vi "SupportedFunctions.vi"(11 "Functions":T1=[{"module"="pyVI.FP.lvFrontPanel", "short name"="", "docstrings"={"type"="def", "name"="_async_raise", "docstring"="raises the exception, performs cleanup if needed"}}, {"module"="pyVI.FP.lvFrontPanel", "short name"="", "docstrings"={"type"="def", "name"="_get_my_tid", "docstring"="determines this (self's) thread id"}}, {"module"="pyVI.FP.lvFrontPanel", "short name"="", "docstrings"={"type"="def", "name"="raise_exc", "docstring"="raises the given exception type in the context of this thread"}}, {"module"="pyVI.FP.lvFrontPanel", "short name"="", "docstrings"={"type"="def", "name"="terminate", "docstring"="raises SystemExit in the context of the given thread, which should \r\n        cause the thread to exit silently (unless caught)"}}, {"module"="pyVI.functions.lvAdvancedFileFunctions", "short name"="lvAdvFile", "docstrings"={"type"="class", "name"="GetFilePosition", "docstring"="_LV_(Get File Position,[1,0],[2,1,0])"}}, {"module"="pyVI.functions.lvAdvancedFileFunctions", "short name"="lvAdvFile", "docstrings"={"type"="class", "name"="GetFileSize", "docstring"="_LV_(Get File Size,[1,0],[2,1,0])"}}, {"module"="pyVI.functions.lvAdvancedFileFunctions", "short name"="lvAdvFile", "docstrings"={"type"="class", "name"="SetFileSize", "docstring"="_LV_(Set File Size,[2,1,0],[1,0])"}}, {"module"="pyVI.functions.lvAdvancedFileFunctions", "short name"="lvAdvFile", "docstrings"={"type"="class", "name"="SetFilePosition", "docstring"="_LV_(Set File Position,[3,2,1,0],[1,0])"}}, {"module"="pyVI.functions.lvAdvancedFileFunctions", "short name"="lvAdvFile", "docstrings"={"type"="class", "name"="MoveFile", "docstring"="_LV_(Move,[4,3,2,0,1],[2,1,0])"}}, {"module"="pyVI.functions.lvAdvancedFileFunctions", "short name"="lvAdvFile", "docstrings"={"type"="class", "name"="CopyFile", "docstring"="_LV_(Copy,[4,3,2,0,1],[2,1,0])"}}, {"module"="pyVI.functions.lvAdvancedFileFunctions", "short name"="lvAdvFile", "docstrings"={"type"="class", "name"="DeleteFile", "docstring"="_LV_(Delete,[4,3,2,0,1],[2,1,0])"}}, {"module"="pyVI.functions.lvAdvancedFileFunctions", "short name"="lvAdvFile", "docstrings"={"type"="class", "name"="CreateFolder", "docstring"="_LV_(Create Folder,[2,0,1],[2,1,0])"}}, {"module"="pyVI.functions.lvAdvancedFileFunctions", "short name"="lvAdvFile", "docstrings"={"type"="class", "name"="ListFolder", "docstring"="_LV_(List Folder,[3,1,0,2],[3,2,1,0])"}}, {"module"="pyVI.functions.lvAdvancedFileFunctions", "short name"="lvAdvFile", "docstrings"={"type"="class", "name"="RefnumToPath", "docstring"="_LV_(Refnum to Path,[0],[0])"}}, {"module"="pyVI.functions.lvAdvancedFileFunctions", "short name"="lvAdvFile", "docstrings"={"type"="class", "name"="PathType", "docstring"="_LV_(Path Type,[0],[0])"}}, {"module"="pyVI.functions.lvArrayFunctions", "short name"="lvArray", "docstrings"={"type"="class", "name"="BuildArray", "docstring"="_LV_(Build Array,[0..],[0])"}}, {"module"="pyVI.functions.lvArrayFunctions", "short name"="lvArray", "docstrings"={"type"="class", "name"="IndexArray", "docstring"="_LV_(Index Array,[0,1..],[0..])"}}, {"module"="pyVI.functions.lvArrayFunctions", "short name"="lvArray", "docstrings"={"type"="class", "name"="ArraySize", "docstring"="_LV_(Array Size,[0],[0])"}}, {"module"="pyVI.functions.lvArrayFunctions", "short name"="lvArray", "docstrings"={"type"="class", "name"="InitializeArray", "docstring"="_LV_(Initialize Array,[0,1..],[0])"}}, {"module"="pyVI.functions.lvArrayFunctions", "short name"="lvArray", "docstrings"={"type"="class", "name"="ArraySubset", "docstring"="_LV_(Array Subset,[0,1,2..],[0])"}}, {"module"="pyVI.functions.lvArrayFunctions", "short name"="lvArray", "docstrings"={"type"="class", "name"="ArrayMaxMin", "docstring"="_LV_(Array Max & Min,[0],[0,1,2,3])"}}, {"module"="pyVI.functions.lvArrayFunctions", "short name"="lvArray", "docstrings"={"type"="class", "name"="ReshapeArray", "docstring"="_LV_(Reshape Array,[0,1..],[0])"}}, {"module"="pyVI.functions.lvArrayFunctions", "short name"="lvArray", "docstrings"={"type"="class", "name"="SortArray", "docstring"="_LV_(Sort 1D Array,[0],[0])"}}, {"module"="pyVI.functions.lvArrayFunctions", "short name"="lvArray", "docstrings"={"type"="class", "name"="SearchArray", "docstring"="_LV_(Search 1D Array,[2,1,0],[0])"}}, {"module"="pyVI.functions.lvArrayFunctions", "short name"="lvArray", "docstrings"={"type"="class", "name"="SplitArray", "docstring"="_LV_(Split 1D Array,[1,0],[1,0])"}}, {"module"="pyVI.functions.lvArrayFunctions", "short name"="lvArray", "docstrings"={"type"="class", "name"="ReverseArray", "docstring"="_LV_(Reverse 1D Array,[0],[0])"}}, {"module"="pyVI.functions.lvArrayFunctions", "short name"="lvArray", "docstrings"={"type"="class", "name"="RotateArray", "docstring"="_LV_(Rotate 1D Array,[0,1],[0])"}}, {"module"="pyVI.functions.lvArrayFunctions", "short name"="lvArray", "docstrings"={"type"="class", "name"="InterleaveArrays", "docstring"="_LV_(Interleave 1D Arrays,[0..],[0])"}}, {"module"="pyVI.functions.lvArrayFunctions", "short name"="lvArray", "docstrings"={"type"="class", "name"="DecimateArray", "docstring"="_LV_(Decimate 1D Array,[0],[0..])"}}, {"module"="pyVI.functions.lvArrayFunctions", "short name"="lvArray", "docstrings"={"type"="class", "name"="TransposeArray", "docstring"="_LV_(Transpose 2D Array,[0],[0])"}}, {"module"="pyVI.functions.lvArrayFunctions", "short name"="lvArray", "docstrings"={"type"="class", "name"="DeleteFromArray", "docstring"="_LV_(Delete From Array,[0,1,2..],[1,0])"}}, {"module"="pyVI.functions.lvArrayFunctions", "short name"="lvArray", "docstrings"={"type"="class", "name"="ReplaceArraySubset", "docstring"="_LV_(Replace Array Subset,[0,1,2..],[0])"}}, {"module"="pyVI.functions.lvArrayFunctions", "short name"="lvArray", "docstrings"={"type"="class", "name"="AddArrayElements", "docstring"="_LV_(Add Array Elements,[0],[0])"}}, {"module"="pyVI.functions.lvArrayFunctions", "short name"="lvArray", "docstrings"={"type"="class", "name"="MultiplyArrayElements", "docstring"="_LV_(Multiply Array Elements,[0],[0])"}}, {"module"="pyVI.functions.lvArrayFunctions", "short name"="lvArray", "docstrings"={"type"="class", "name"="Threshold1DArray", "docstring"="_LV_(Threshold 1D Array,[2,1,0],[0])"}}, {"module"="pyVI.functions.lvArrayFunctions", "short name"="lvArray", "docstrings"={"type"="class", "name"="Interpolate1DArray", "docstring"="_LV_(Interpolate 1D Array,[1,0],[0])"}}, {"module"="pyVI.functions.lvBooleanFunctions", "short name"="lvBool", "docstrings"={"type"="class", "name"="And", "docstring"="_LV_(And,[1,0],[0])"}}, {"module"="pyVI.functions.lvBooleanFunctions", "short name"="lvBool", "docstrings"={"type"="class", "name"="Or", "docstring"="_LV_(Or,[1,0],[0])"}}, {"module"="pyVI.functions.lvBooleanFunctions", "short name"="lvBool", "docstrings"={"type"="class", "name"="Xor", "docstring"="_LV_(Exclusive Or,[1,0],[0])"}}, {"module"="pyVI.functions.lvBooleanFunctions", "short name"="lvBool", "docstrings"={"type"="class", "name"="Not", "docstring"="_LV_(Not,[0],[0])"}}, {"module"="pyVI.functions.lvBooleanFunctions", "short name"="lvBool", "docstrings"={"type"="class", "name"="Nand", "docstring"="_LV_(Not And,[1,0],[0])"}}, {"module"="pyVI.functions.lvBooleanFunctions", "short name"="lvBool", "docstrings"={"type"="class", "name"="Nor", "docstring"="_LV_(Not Or,[1,0],[0])"}}, {"module"="pyVI.functions.lvBooleanFunctions", "short name"="lvBool", "docstrings"={"type"="class", "name"="Nxor", "docstring"="_LV_(Not Exclusive Or,[1,0],[0])"}}, {"module"="pyVI.functions.lvBooleanFunctions", "short name"="lvBool", "docstrings"={"type"="class", "name"="Implies", "docstring"="_LV_(Implies,[1,0],[0])"}}, {"module"="pyVI.functions.lvBooleanFunctions", "short name"="lvBool", "docstrings"={"type"="class", "name"="And_array_elements", "docstring"="_LV_(And Array Elements,[0],[0])"}}, {"module"="pyVI.functions.lvBooleanFunctions", "short name"="lvBool", "docstrings"={"type"="class", "name"="Or_array_elements", "docstring"="_LV_(Or Array Elements,[0],[0])"}}, {"module"="pyVI.functions.lvBooleanFunctions", "short name"="lvBool", "docstrings"={"type"="class", "name"="Number_to_boolean_array", "docstring"="_LV_(Number To Boolean Array,[0],[0])"}}, {"module"="pyVI.functions.lvBooleanFunctions", "short name"="lvBool", "docstrings"={"type"="class", "name"="Boolean_to_0_1", "docstring"="_LV_(Boolean To (0,1),[0],[0])"}}, {"module"="pyVI.functions.lvClusterFunctions", "short name"="lvClust", "docstrings"={"type"="class", "name"="UnbundleByName", "docstring"="_LV_(Unbundle By Name,[0],[0..])"}}, {"module"="pyVI.functions.lvClusterFunctions", "short name"="lvClust", "docstrings"={"type"="class", "name"="Unbundle", "docstring"="_LV_(Unbundle,[0],[0..])"}}, {"module"="pyVI.functions.lvClusterFunctions", "short name"="lvClust", "docstrings"={"type"="class", "name"="BundleByName", "docstring"="_LV_(Bundle By Name,[0..],[0])"}}, {"module"="pyVI.functions.lvClusterFunctions", "short name"="lvClust", "docstrings"={"type"="class", "name"="Bundle", "docstring"="_LV_(Bundle,[0..],[0])"}}, {"module"="pyVI.functions.lvComparisons", "short name"="lvComp", "docstrings"={"type"="class", "name"="Equals", "docstring"="_LV_(Equal?,[1,0],[0])"}}, {"module"="pyVI.functions.lvComparisons", "short name"="lvComp", "docstrings"={"type"="class", "name"="NotEquals", "docstring"="_LV_(Not Equal?,[1,0],[0])"}}, {"module"="pyVI.functions.lvComparisons", "short name"="lvComp", "docstrings"={"type"="class", "name"="GreaterThan", "docstring"="_LV_(Greater?,[1,0],[0])"}}, {"module"="pyVI.functions.lvComparisons", "short name"="lvComp", "docstrings"={"type"="class", "name"="GreaterThanOrEqual", "docstring"="_LV_(Greater Or Equal?,[1,0],[0])"}}, {"module"="pyVI.functions.lvComparisons", "short name"="lvComp", "docstrings"={"type"="class", "name"="LessThan", "docstring"="_LV_(Less?,[1,0],[0])"}}, {"module"="pyVI.functions.lvComparisons", "short name"="lvComp", "docstrings"={"type"="class", "name"="LessThanOrEqual", "docstring"="_LV_(Less Or Equal?,[1,0],[0])"}}, {"module"="pyVI.functions.lvComparisons", "short name"="lvComp", "docstrings"={"type"="class", "name"="EqualZero", "docstring"="_LV_(Equal To 0?,[0],[0])"}}, {"module"="pyVI.functions.lvComparisons", "short name"="lvComp", "docstrings"={"type"="class", "name"="NotEqualZero", "docstring"="_LV_(Not Equal To 0?,[0],[0])"}}, {"module"="pyVI.functions.lvComparisons", "short name"="lvComp", "docstrings"={"type"="class", "name"="GreaterThanZero", "docstring"="_LV_(Greater Than 0?,[0],[0])"}}, {"module"="pyVI.functions.lvComparisons", "short name"="lvComp", "docstrings"={"type"="class", "name"="GreaterThanOrEqualToZero", "docstring"="_LV_(Greater Or Equal To 0?,[0],[0])"}}, {"module"="pyVI.functions.lvComparisons", "short name"="lvComp", "docstrings"={"type"="class", "name"="LessThanZero", "docstring"="_LV_(Less Than 0?,[0],[0])"}}, {"module"="pyVI.functions.lvComparisons", "short name"="lvComp", "docstrings"={"type"="class", "name"="LessThanOrEqualToZero", "docstring"="_LV_(Less Or Equal To 0?,[0],[0])"}}, {"module"="pyVI.functions.lvComparisons", "short name"="lvComp", "docstrings"={"type"="class", "name"="MaxMin", "docstring"="_LV_(Max & Min,[1,0],[1,0])"}}, {"module"="pyVI.functions.lvComparisons", "short name"="lvComp", "docstrings"={"type"="class", "name"="Select", "docstring"="_LV_(Select,[1,2,0],[0])"}}, {"module"="pyVI.functions.lvComparisons", "short name"="lvComp", "docstrings"={"type"="class", "name"="EmptyArray", "docstring"="_LV_(Empty Array?,[0],[0])"}}, {"module"="pyVI.functions.lvComparisons", "short name"="lvComp", "docstrings"={"type"="class", "name"="EmptyString", "docstring"="_LV_(Empty String/Path?,[0],[0])"}}, {"module"="pyVI.functions.lvComparisons", "short name"="lvComp", "docstrings"={"type"="class", "name"="NotANumber", "docstring"="_LV_(Not A Number/Path/Refnum?,[0],[0])"}}, {"module"="pyVI.functions.lvComparisons", "short name"="lvComp", "docstrings"={"type"="class", "name"="InRangeAndCoerce", "docstring"="_LV_(In Range and Coerce,[2,1,0],[1,0])"}}, {"module"="pyVI.functions.lvComparisons", "short name"="lvComp", "docstrings"={"type"="class", "name"="LexicalClass", "docstring"="_LV_(Lexical Class,[0],[0])"}}, {"module"="pyVI.functions.lvDataManipulation", "short name"="lvDataMan", "docstrings"={"type"="class", "name"="TypeCast", "docstring"="_LV_(Type Cast,[0,1],[0])"}}, {"module"="pyVI.functions.lvDataManipulation", "short name"="lvDataMan", "docstrings"={"type"="class", "name"="SplitNumber", "docstring"="_LV_(Split Number,[0],[1,0])"}}, {"module"="pyVI.functions.lvDataManipulation", "short name"="lvDataMan", "docstrings"={"type"="class", "name"="JoinNumbers", "docstring"="_LV_(Join Numbers,[0,1],[0])"}}, {"module"="pyVI.functions.lvDataManipulation", "short name"="lvDataMan", "docstrings"={"type"="class", "name"="SwapBytes", "docstring"="_LV_(Swap Bytes,[0],[0])"}}, {"module"="pyVI.functions.lvDataManipulation", "short name"="lvDataMan", "docstrings"={"type"="class", "name"="SwapWords", "docstring"="_LV_(Swap Words,[0],[0])"}}, {"module"="pyVI.functions.lvDataManipulation", "short name"="lvDataMan", "docstrings"={"type"="class", "name"="RotateLeftWithCarry", "docstring"="_LV_(Rotate Left With Carry,[0,1],[0,1])"}}, {"module"="pyVI.functions.lvDataManipulation", "short name"="lvDataMan", "docstrings"={"type"="class", "name"="RotateRightWithCarry", "docstring"="_LV_(Rotate Right With Carry,[0,1],[0,1])"}}, {"module"="pyVI.functions.lvDataManipulation", "short name"="lvDataMan", "docstrings"={"type"="class", "name"="LogicalShift", "docstring"="_LV_(Logical Shift,[0,1],[0])"}}, {"module"="pyVI.functions.lvDataManipulation", "short name"="lvDataMan", "docstrings"={"type"="class", "name"="Rotate", "docstring"="_LV_(Rotate,[0,1],[0])"}}, {"module"="pyVI.functions.lvDataManipulation", "short name"="lvDataMan", "docstrings"={"type"="class", "name"="FlattenToString", "docstring"="_LV_(Flatten To String,[3,2,1,0],[2,0])"}}, {"module"="pyVI.functions.lvDataManipulation", "short name"="lvDataMan", "docstrings"={"type"="class", "name"="UnflattenFromString", "docstring"="_LV_(Unflatten From String,[4,0,3,2,1],[2,1,0])"}}, {"module"="pyVI.functions.lvDataManipulation", "short name"="lvDataMan", "docstrings"={"type"="class", "name"="MantissaAndExponent", "docstring"="_LV_(Mantissa & Exponent,[0],[0,1])"}}, {"module"="pyVI.functions.lvDialog", "short name"="lvDialog", "docstrings"={"type"="class", "name"="lvOneButtonDialog", "docstring"="_LV_(One Button Dialog,[1,0],[0])"}}, {"module"="pyVI.functions.lvDialog", "short name"="lvDialog", "docstrings"={"type"="class", "name"="lvTwoButtonDialog", "docstring"="_LV_(Two Button Dialog,[2,1,0],[0])"}}, {"module"="pyVI.functions.lvDialog", "short name"="lvDialog", "docstrings"={"type"="class", "name"="ClearErrors", "docstring"="_LV_(Clear Errors.vi,[1,0],[1,0])"}}, {"module"="pyVI.functions.lvDialog", "short name"="lvDialog", "docstrings"={"type"="class", "name"="MergeErrors", "docstring"="_LV_(Merge Errors,[0..],[0])"}}, {"module"="pyVI.functions.lvDialog", "short name"="lvDialog", "docstrings"={"type"="class", "name"="SimpleErrorHandler", "docstring"="_LV_(Simple Error Handler.vi,[0,1,2,3],[0,1,2,4,3])"}}, {"module"="pyVI.functions.lvDialog", "short name"="lvDialog", "docstrings"={"type"="class", "name"="WaitForFrontPanelActivity", "docstring"="_LV_(Wait For Front Panel Activity,[2,1,0],[0])"}}, {"module"="pyVI.functions.lvExponentialFunctions", "short name"="lvExp", "docstrings"={"type"="class", "name"="Exp", "docstring"="_LV_(Exponential,[0],[0])"}}, {"module"="pyVI.functions.lvExponentialFunctions", "short name"="lvExp", "docstrings"={"type"="class", "name"="Exp_minus_1", "docstring"="_LV_(Exponential (Arg) -1,[0],[0])"}}, {"module"="pyVI.functions.lvExponentialFunctions", "short name"="lvExp", "docstrings"={"type"="class", "name"="Power_of_2", "docstring"="_LV_(Power Of 2,[0],[0])"}}, {"module"="pyVI.functions.lvExponentialFunctions", "short name"="lvExp", "docstrings"={"type"="class", "name"="Power_of_X", "docstring"="_LV_(Power Of X,[0,1],[0])"}}, {"module"="pyVI.functions.lvExponentialFunctions", "short name"="lvExp", "docstrings"={"type"="class", "name"="Ln", "docstring"="_LV_(Natural Logarithm,[0],[0])"}}, {"module"="pyVI.functions.lvExponentialFunctions", "short name"="lvExp", "docstrings"={"type"="class", "name"="Log10", "docstring"="_LV_(Logarithm Base 10,[0],[0])"}}, {"module"="pyVI.functions.lvExponentialFunctions", "short name"="lvExp", "docstrings"={"type"="class", "name"="Log2", "docstring"="_LV_(Logarithm Base 2,[0],[0])"}}, {"module"="pyVI.functions.lvFileFunctions", "short name"="lvFile", "docstrings"={"type"="class", "name"="BuildPath", "docstring"="_LV_(Build Path,[1,0],[0])"}}, {"module"="pyVI.functions.lvFileFunctions", "short name"="lvFile", "docstrings"={"type"="class", "name"="StripPath", "docstring"="_LV_(Strip Path,[0],[0,1])"}}, {"module"="pyVI.functions.lvFileFunctions", "short name"="lvFile", "docstrings"={"type"="class", "name"="ReadFromTextFile", "docstring"="_LV_(Read from Text File,[3,2,0,1],[3,2,1,0])"}}, {"module"="pyVI.functions.lvFileFunctions", "short name"="lvFile", "docstrings"={"type"="class", "name"="WriteToTextFile", "docstring"="_LV_(Write to Text File,[3,2,0,1],[2,1,0])"}}, {"module"="pyVI.functions.lvFileFunctions", "short name"="lvFile", "docstrings"={"type"="class", "name"="OpenFile", "docstring"="_LV_(Open/Create/Replace File,[5,4,3,1,0,2],[2,1,0])"}}, {"module"="pyVI.functions.lvFileFunctions", "short name"="lvFile", "docstrings"={"type"="class", "name"="CloseFile", "docstring"="_LV_(Close File,[1,0],[1,0])"}}, {"module"="pyVI.functions.lvHyperbolicFunctions", "short name"="lvHyper", "docstrings"={"type"="class", "name"="Hyperbolic_sine", "docstring"="_LV_(Hyperbolic Sine,[0],[0])"}}, {"module"="pyVI.functions.lvHyperbolicFunctions", "short name"="lvHyper", "docstrings"={"type"="class", "name"="Hyperbolic_cosine", "docstring"="_LV_(Hyperbolic Cosine,[0],[0])"}}, {"module"="pyVI.functions.lvHyperbolicFunctions", "short name"="lvHyper", "docstrings"={"type"="class", "name"="Hyperbolic_tangent", "docstring"="_LV_(Hyperbolic Tangent,[0],[0])"}}, {"module"="pyVI.functions.lvHyperbolicFunctions", "short name"="lvHyper", "docstrings"={"type"="class", "name"="Arc_Hyperbolic_sine", "docstring"="_LV_(Inverse Hyperbolic Sine,[0],[0])"}}, {"module"="pyVI.functions.lvHyperbolicFunctions", "short name"="lvHyper", "docstrings"={"type"="class", "name"="Arc_Hyperbolic_cosine", "docstring"="_LV_(Inverse Hyperbolic Cosine,[0],[0])"}}, {"module"="pyVI.functions.lvHyperbolicFunctions", "short name"="lvHyper", "docstrings"={"type"="class", "name"="Arc_Hyperbolic_tangent", "docstring"="_LV_(Inverse Hyperbolic Tangent,[0],[0])"}}, {"module"="pyVI.functions.lvHyperbolicFunctions", "short name"="lvHyper", "docstrings"={"type"="class", "name"="Hyperbolic_secant", "docstring"="_LV_(Hyperbolic Secant,[0],[0])"}}, {"module"="pyVI.functions.lvHyperbolicFunctions", "short name"="lvHyper", "docstrings"={"type"="class", "name"="Arc_Hyperbolic_secant", "docstring"="_LV_(Inverse Hyperbolic Secant,[0],[0])"}}, {"module"="pyVI.functions.lvHyperbolicFunctions", "short name"="lvHyper", "docstrings"={"type"="class", "name"="Hyperbolic_cosecant", "docstring"="_LV_(Hyperbolic Cosecant,[0],[0])"}}, {"module"="pyVI.functions.lvHyperbolicFunctions", "short name"="lvHyper", "docstrings"={"type"="class", "name"="Arc_Hyperbolic_cosecant", "docstring"="_LV_(Inverse Hyperbolic Cosecant,[0],[0])"}}, {"module"="pyVI.functions.lvHyperbolicFunctions", "short name"="lvHyper", "docstrings"={"type"="class", "name"="Hyperbolic_cotangent", "docstring"="_LV_(Hyperbolic Cotangent,[0],[0])"}}, {"module"="pyVI.functions.lvHyperbolicFunctions", "short name"="lvHyper", "docstrings"={"type"="class", "name"="Arc_Hyperbolic_cotangent", "docstring"="_LV_(Inverse Hyperbolic Cotangent,[0],[0])"}}, {"module"="pyVI.functions.lvNetworking", "short name"="lvNet", "docstrings"={"type"="class", "name"="UDPOpen", "docstring"="_LV_(UDP Open,[4,3,2,0,1],[2,1,0])"}}, {"module"="pyVI.functions.lvNetworking", "short name"="lvNet", "docstrings"={"type"="class", "name"="UDPMulticastOpen", "docstring"="_LV_(UDP Multicast Open,[4,3,2,0,1],[2,1,0])"}}, {"module"="pyVI.functions.lvNetworking", "short name"="lvNet", "docstrings"={"type"="class", "name"="UDPMulticastReadOpen", "docstring"="_LV_(#UDP Multicast Read-Only Open.vi,[4,3,2,0,1],[2,1,0])"}}, {"module"="pyVI.functions.lvNetworking", "short name"="lvNet", "docstrings"={"type"="class", "name"="UDPMulticastWriteOpen", "docstring"="_LV_(#UDP Multicast Write-Only Open.vi,[4,3,2,0,1],[2,1,0])"}}, {"module"="pyVI.functions.lvNetworking", "short name"="lvNet", "docstrings"={"type"="class", "name"="UDPMulticastReadWriteOpen", "docstring"="_LV_(#UDP Multicast Read-Write Open.vi,[4,3,2,0,1],[2,1,0])"}}, {"module"="pyVI.functions.lvNetworking", "short name"="lvNet", "docstrings"={"type"="class", "name"="UDPRead", "docstring"="_LV_(UDP Read,[3,2,1,0],[2,1,3,4,0])"}}, {"module"="pyVI.functions.lvNetworking", "short name"="lvNet", "docstrings"={"type"="class", "name"="UDPWrite", "docstring"="_LV_(UDP Write,[5,0,1,4,3,2],[1,0])"}}, {"module"="pyVI.functions.lvNetworking", "short name"="lvNet", "docstrings"={"type"="class", "name"="UDPClose", "docstring"="_LV_(UDP Close,[1,0],[1,0])"}}, {"module"="pyVI.functions.lvNetworking", "short name"="lvNet", "docstrings"={"type"="class", "name"="IPtoString", "docstring"="_LV_(IP To String,[1,0],[0])"}}, {"module"="pyVI.functions.lvNetworking", "short name"="lvNet", "docstrings"={"type"="class", "name"="StringToIP", "docstring"="_LV_(String To IP,[0],[0])"}}, {"module"="pyVI.functions.lvNetworking", "short name"="lvNet", "docstrings"={"type"="class", "name"="TCPOpen", "docstring"="_LV_(TCP Open Connection,[3,4,2,0,1],[1,0])"}}, {"module"="pyVI.functions.lvNetworking", "short name"="lvNet", "docstrings"={"type"="class", "name"="TCPClose", "docstring"="_LV_(TCP Close Connection,[2,1,0],[1,0])"}}, {"module"="pyVI.functions.lvNetworking", "short name"="lvNet", "docstrings"={"type"="class", "name"="TCPRead", "docstring"="_LV_(TCP Read,[4,3,2,0,1],[2,1,0])"}}, {"module"="pyVI.functions.lvNetworking", "short name"="lvNet", "docstrings"={"type"="class", "name"="TCPWrite", "docstring"="_LV_(TCP Write,[3,2,1,0],[2,1,0])"}}, {"module"="pyVI.functions.lvNetworking", "short name"="lvNet", "docstrings"={"type"="class", "name"="TCPCreateListener", "docstring"="_LV_(TCP Create Listener,[3,4,2,0,1],[2,1,0])"}}, {"module"="pyVI.functions.lvNetworking", "short name"="lvNet", "docstrings"={"type"="class", "name"="TCPWaitOnListener", "docstring"="_LV_(TCP Wait On Listener,[3,2,1,0],[3,2,1,4,0])"}}, {"module"="pyVI.functions.lvNumericConversion", "short name"="lvNumConv", "docstrings"={"type"="class", "name"="toDBL", "docstring"="_LV_(To Double Precision Float,[0],[0])"}}, {"module"="pyVI.functions.lvNumericConversion", "short name"="lvNumConv", "docstrings"={"type"="class", "name"="toSGL", "docstring"="_LV_(To Single Precision Float,[0],[0])"}}, {"module"="pyVI.functions.lvNumericConversion", "short name"="lvNumConv", "docstrings"={"type"="class", "name"="toEXT", "docstring"="_LV_(To Extended Precision Float,[0],[0])"}}, {"module"="pyVI.functions.lvNumericConversion", "short name"="lvNumConv", "docstrings"={"type"="class", "name"="toU64", "docstring"="_LV_(To Unsigned Quad Integer,[0],[0])"}}, {"module"="pyVI.functions.lvNumericConversion", "short name"="lvNumConv", "docstrings"={"type"="class", "name"="toU32", "docstring"="_LV_(To Unsigned Long Integer,[0],[0])"}}, {"module"="pyVI.functions.lvNumericConversion", "short name"="lvNumConv", "docstrings"={"type"="class", "name"="toU16", "docstring"="_LV_(To Unsigned Word Integer,[0],[0])"}}, {"module"="pyVI.functions.lvNumericConversion", "short name"="lvNumConv", "docstrings"={"type"="class", "name"="toU8", "docstring"="_LV_(To Unsigned Byte Integer,[0],[0])"}}, {"module"="pyVI.functions.lvNumericConversion", "short name"="lvNumConv", "docstrings"={"type"="class", "name"="toI64", "docstring"="_LV_(To Quad Integer,[0],[0])"}}, {"module"="pyVI.functions.lvNumericConversion", "short name"="lvNumConv", "docstrings"={"type"="class", "name"="toI32", "docstring"="_LV_(To Long Integer,[0],[0])"}}, {"module"="pyVI.functions.lvNumericConversion", "short name"="lvNumConv", "docstrings"={"type"="class", "name"="toI16", "docstring"="_LV_(To Word Integer,[0],[0])"}}, {"module"="pyVI.functions.lvNumericConversion", "short name"="lvNumConv", "docstrings"={"type"="class", "name"="toI8", "docstring"="_LV_(To Byte Integer,[0],[0])"}}, {"module"="pyVI.functions.lvNumericConversion", "short name"="lvNumConv", "docstrings"={"type"="class", "name"="toTimestamp", "docstring"="_LV_(To Time Stamp,[0],[0])"}}, {"module"="pyVI.functions.lvNumericFunctions", "short name"="lvNum", "docstrings"={"type"="class", "name"="Add", "docstring"="_LV_(Add,[1,0],[0])"}}, {"module"="pyVI.functions.lvNumericFunctions", "short name"="lvNum", "docstrings"={"type"="class", "name"="Subtract", "docstring"="_LV_(Subtract,[1,0],[0])"}}, {"module"="pyVI.functions.lvNumericFunctions", "short name"="lvNum", "docstrings"={"type"="class", "name"="Multiply", "docstring"="_LV_(Multiply,[1,0],[0])"}}, {"module"="pyVI.functions.lvNumericFunctions", "short name"="lvNum", "docstrings"={"type"="class", "name"="Divide", "docstring"="_LV_(Divide,[1,0],[0])"}}, {"module"="pyVI.functions.lvNumericFunctions", "short name"="lvNum", "docstrings"={"type"="class", "name"="Abs", "docstring"="_LV_(Absolute Value,[0],[0])"}}, {"module"="pyVI.functions.lvNumericFunctions", "short name"="lvNum", "docstrings"={"type"="class", "name"="Round", "docstring"="_LV_(Round To Nearest,[0],[0])"}}, {"module"="pyVI.functions.lvNumericFunctions", "short name"="lvNum", "docstrings"={"type"="class", "name"="Round_plus_infinity", "docstring"="_LV_(Round Toward +Infinity,[0],[0])"}}, {"module"="pyVI.functions.lvNumericFunctions", "short name"="lvNum", "docstrings"={"type"="class", "name"="Round_minus_infinity", "docstring"="_LV_(Round Toward -Infinity,[0],[0])"}}, {"module"="pyVI.functions.lvNumericFunctions", "short name"="lvNum", "docstrings"={"type"="class", "name"="SquareRoot", "docstring"="_LV_(Square Root,[0],[0])"}}, {"module"="pyVI.functions.lvNumericFunctions", "short name"="lvNum", "docstrings"={"type"="class", "name"="Square", "docstring"="_LV_(Square,[0],[0])"}}, {"module"="pyVI.functions.lvNumericFunctions", "short name"="lvNum", "docstrings"={"type"="class", "name"="Negate", "docstring"="_LV_(Negate,[0],[0])"}}, {"module"="pyVI.functions.lvNumericFunctions", "short name"="lvNum", "docstrings"={"type"="class", "name"="Reciprocal", "docstring"="_LV_(Reciprocal,[0],[0])"}}, {"module"="pyVI.functions.lvNumericFunctions", "short name"="lvNum", "docstrings"={"type"="class", "name"="Sign", "docstring"="_LV_(Sign,[0],[0])"}}, {"module"="pyVI.functions.lvNumericFunctions", "short name"="lvNum", "docstrings"={"type"="class", "name"="Random", "docstring"="_LV_(Random Number (0-1),[],[0])"}}, {"module"="pyVI.functions.lvNumericFunctions", "short name"="lvNum", "docstrings"={"type"="class", "name"="Quotient_and_Remainder", "docstring"="_LV_(Quotient & Remainder,[1,0],[1,0])"}}, {"module"="pyVI.functions.lvNumericFunctions", "short name"="lvNum", "docstrings"={"type"="class", "name"="Increment", "docstring"="_LV_(Increment,[0],[0])"}}, {"module"="pyVI.functions.lvNumericFunctions", "short name"="lvNum", "docstrings"={"type"="class", "name"="Decrement", "docstring"="_LV_(Decrement,[0],[0])"}}, {"module"="pyVI.functions.lvNumericFunctions", "short name"="lvNum", "docstrings"={"type"="class", "name"="CompoundArithmetic", "docstring"="_LV_(Compound Arithmetic,[0..],[0])"}}, {"module"="pyVI.functions.lvNumericFunctions", "short name"="lvNum", "docstrings"={"type"="class", "name"="ScaleByPowerOf2", "docstring"="_LV_(Scale By Power Of 2,[1,0],[0])"}}, {"module"="pyVI.functions.lvProbabilityAndStatistics", "short name"="lvProbStats", "docstrings"={"type"="class", "name"="Mean_DBL", "docstring"="_LV_(NI_AALBase.lvlib:Mean (DBL).vi,[0],[0,1])"}}, {"module"="pyVI.functions.lvProbabilityAndStatistics", "short name"="lvProbStats", "docstrings"={"type"="class", "name"="Std_Deviation_and_Variance", "docstring"="_LV_(NI_AALBase.lvlib:Std Deviation and Variance.vi,[0,1],[0,1,2])"}}, {"module"="pyVI.functions.lvProbabilityAndStatistics", "short name"="lvProbStats", "docstrings"={"type"="class", "name"="Median", "docstring"="_LV_(NI_AALBase.lvlib:Median.vi,[0],[0,1])"}}, {"module"="pyVI.functions.lvProbabilityAndStatistics", "short name"="lvProbStats", "docstrings"={"type"="class", "name"="RMS_DBL", "docstring"="_LV_(NI_AALPro.lvlib:RMS (DBL).vi,[0],[0,1])"}}, {"module"="pyVI.functions.lvQueueFunctions", "short name"="lvQueue", "docstrings"={"type"="class", "name"="ObtainQueue", "docstring"="_LV_(Obtain Queue,[0,1,2,4,3],[0,1,2])"}}, {"module"="pyVI.functions.lvQueueFunctions", "short name"="lvQueue", "docstrings"={"type"="class", "name"="EnqueueElement", "docstring"="_LV_(Enqueue Element,[0,1,2,3],[0,1,2])"}}, {"module"="pyVI.functions.lvQueueFunctions", "short name"="lvQueue", "docstrings"={"type"="class", "name"="EnqueueElementAtOppositeEnd", "docstring"="_LV_(Enqueue Element At Opposite End,[0,1,2,3],[0,1,2])"}}, {"module"="pyVI.functions.lvQueueFunctions", "short name"="lvQueue", "docstrings"={"type"="class", "name"="LossyEnqueueElement", "docstring"="_LV_(Lossy Enqueue Element,[0,1,2],[0,1,2])"}}, {"module"="pyVI.functions.lvQueueFunctions", "short name"="lvQueue", "docstrings"={"type"="class", "name"="DequeueElement", "docstring"="_LV_(Dequeue Element,[0,1,2],[0,1,2,3])"}}, {"module"="pyVI.functions.lvQueueFunctions", "short name"="lvQueue", "docstrings"={"type"="class", "name"="FlushQueue", "docstring"="_LV_(Flush Queue,[0,1],[0,1,2])"}}, {"module"="pyVI.functions.lvQueueFunctions", "short name"="lvQueue", "docstrings"={"type"="class", "name"="ReleaseQueue", "docstring"="_LV_(Release Queue,[0,1,2],[0,1,2])"}}, {"module"="pyVI.functions.lvSignalOperations", "short name"="lvSigOp", "docstrings"={"type"="class", "name"="Peak_Detector", "docstring"="_LV_(NI_AAL_SigProc.lvlib:Peak Detector.vi,[5,3,4,2,1,0],[4,3,2,1,0])"}}, {"module"="pyVI.functions.lvSignalOperations", "short name"="lvSigOp", "docstrings"={"type"="class", "name"="Scaled_Time_Domain_Window_DBL", "docstring"="_LV_(NI_AALPro.lvlib:Scaled Time Domain Window (DBL).vi,[2,1,0],[2,1,0])"}}, {"module"="pyVI.functions.lvSignalOperations", "short name"="lvSigOp", "docstrings"={"type"="class", "name"="Power_Spectrum_DBL", "docstring"="_LV_(NI_AALPro.lvlib:Power Spectrum (DBL).vi,[0],[0,1])"}}, {"module"="pyVI.functions.lvSignalOperations", "short name"="lvSigOp", "docstrings"={"type"="class", "name"="Decimate_continuous_DBL", "docstring"="_LV_(NI_AALPro.lvlib:Decimate (continuous, DBL).vi,[5,4,3,0,1,2],[1,0])"}}, {"module"="pyVI.functions.lvStringArrayPathConversion", "short name"="lvStrArrPath", "docstrings"={"type"="class", "name"="StringToByteArray", "docstring"="_LV_(String To Byte Array,[0],[0])"}}, {"module"="pyVI.functions.lvStringArrayPathConversion", "short name"="lvStrArrPath", "docstrings"={"type"="class", "name"="ByteArrayToString", "docstring"="_LV_(Byte Array To String,[0],[0])"}}, {"module"="pyVI.functions.lvStringArrayPathConversion", "short name"="lvStrArrPath", "docstrings"={"type"="class", "name"="PathToArrayOfStrings", "docstring"="_LV_(Path to Array of Strings,[0],[1,0])"}}, {"module"="pyVI.functions.lvStringArrayPathConversion", "short name"="lvStrArrPath", "docstrings"={"type"="class", "name"="ArrayOfStringsToPath", "docstring"="_LV_(Array of Strings To Path,[0,1],[0])"}}, {"module"="pyVI.functions.lvStringArrayPathConversion", "short name"="lvStrArrPath", "docstrings"={"type"="class", "name"="PathToString", "docstring"="_LV_(Path To String,[0],[0])"}}, {"module"="pyVI.functions.lvStringArrayPathConversion", "short name"="lvStrArrPath", "docstrings"={"type"="class", "name"="StringToPath", "docstring"="_LV_(String To Path,[0],[0])"}}, {"module"="pyVI.functions.lvStringFunctions", "short name"="lvStr", "docstrings"={"type"="class", "name"="StringLength", "docstring"="_LV_(String Length,[0],[0])"}}, {"module"="pyVI.functions.lvStringFunctions", "short name"="lvStr", "docstrings"={"type"="class", "name"="ConcatenateStrings", "docstring"="_LV_(Concatenate Strings,[0..],[0])"}}, {"module"="pyVI.functions.lvStringFunctions", "short name"="lvStr", "docstrings"={"type"="class", "name"="StringSubset", "docstring"="_LV_(String Subset,[2,1,0],[0])"}}, {"module"="pyVI.functions.lvStringFunctions", "short name"="lvStr", "docstrings"={"type"="class", "name"="ReplaceSubstring", "docstring"="_LV_(Replace Substring,[3,2,1,0],[1,0])"}}, {"module"="pyVI.functions.lvStringFunctions", "short name"="lvStr", "docstrings"={"type"="class", "name"="TrimWhitespace", "docstring"="_LV_(Trim Whitespace.vi,[0,1],[0])"}}, {"module"="pyVI.functions.lvStringFunctions", "short name"="lvStr", "docstrings"={"type"="class", "name"="ToUpperCase", "docstring"="_LV_(To Upper Case,[0],[0])"}}, {"module"="pyVI.functions.lvStringFunctions", "short name"="lvStr", "docstrings"={"type"="class", "name"="ToLowerCase", "docstring"="_LV_(To Lower Case,[0],[0])"}}, {"module"="pyVI.functions.lvStringFunctions", "short name"="lvStr", "docstrings"={"type"="class", "name"="ArrayToSpreadsheetString", "docstring"="_LV_(Array To Spreadsheet String,[1,2,0],[0])"}}, {"module"="pyVI.functions.lvStringFunctions", "short name"="lvStr", "docstrings"={"type"="class", "name"="SpreadsheetStringToArray", "docstring"="_LV_(Spreadsheet String To Array,[2,3,0,1],[0])"}}, {"module"="pyVI.functions.lvStringFunctions", "short name"="lvStr", "docstrings"={"type"="class", "name"="MatchPattern", "docstring"="_LV_(Match Pattern,[0,1,2],[0,1,2,3])"}}, {"module"="pyVI.functions.lvStringFunctions", "short name"="lvStr", "docstrings"={"type"="class", "name"="SearchAndReplaceString", "docstring"="_LV_(Search and Replace String,[0,4,5,6,1,2,3,7],[0,1,2,3])"}}, {"module"="pyVI.functions.lvStringFunctions", "short name"="lvStr", "docstrings"={"type"="class", "name"="FormatIntoString", "docstring"="_LV_(Format Into String,[0,1,2..],[0,1])"}}, {"module"="pyVI.functions.lvStringFunctions", "short name"="lvStr", "docstrings"={"type"="class", "name"="ScanFromString", "docstring"="_LV_(Scan From String,[0,1,2,3..],[0,1,2,3..])"}}, {"module"="pyVI.functions.lvStringNumberConversions", "short name"="lvStrConv", "docstrings"={"type"="class", "name"="NumberToDecimalString", "docstring"="_LV_(Number To Decimal String,[1,0],[0])"}}, {"module"="pyVI.functions.lvStringNumberConversions", "short name"="lvStrConv", "docstrings"={"type"="class", "name"="NumberToHexString", "docstring"="_LV_(Number To Hexadecimal String,[1,0],[0])"}}, {"module"="pyVI.functions.lvStringNumberConversions", "short name"="lvStrConv", "docstrings"={"type"="class", "name"="NumberToOctalString", "docstring"="_LV_(Number To Octal String,[1,0],[0])"}}, {"module"="pyVI.functions.lvStringNumberConversions", "short name"="lvStrConv", "docstrings"={"type"="class", "name"="NumberToFractionalString", "docstring"="_LV_(Number To Fractional String,[3,2,1,0],[0])"}}, {"module"="pyVI.functions.lvStringNumberConversions", "short name"="lvStrConv", "docstrings"={"type"="class", "name"="NumberToExpString", "docstring"="_LV_(Number To Exponential String,[3,1,2,0],[0])"}}, {"module"="pyVI.functions.lvStringNumberConversions", "short name"="lvStrConv", "docstrings"={"type"="class", "name"="FormatValue", "docstring"="_LV_(Format Value,[0,1,2],[0])"}}, {"module"="pyVI.functions.lvStringNumberConversions", "short name"="lvStrConv", "docstrings"={"type"="class", "name"="DecimalStringToNumber", "docstring"="_LV_(Decimal String To Number,[2,1,0],[0,1])"}}, {"module"="pyVI.functions.lvStringNumberConversions", "short name"="lvStrConv", "docstrings"={"type"="class", "name"="HexadecimalStringToNumber", "docstring"="_LV_(Hexadecimal String To Number,[2,1,0],[0,1])"}}, {"module"="pyVI.functions.lvStringNumberConversions", "short name"="lvStrConv", "docstrings"={"type"="class", "name"="OctalStringToNumber", "docstring"="_LV_(Octal String To Number,[2,1,0],[0,1])"}}, {"module"="pyVI.functions.lvStringNumberConversions", "short name"="lvStrConv", "docstrings"={"type"="class", "name"="FractionalStringToNumber", "docstring"="_LV_(Fract/Exp String To Number,[3,2,1,0],[0,1])"}}, {"module"="pyVI.functions.lvSynchronization", "short name"="lvSync", "docstrings"={"type"="class", "name"="FirstCall", "docstring"="_LV_(First Call?,[],[0])"}}, {"module"="pyVI.functions.lvTimeFunctions", "short name"="lvTiming", "docstrings"={"type"="class", "name"="tickCount", "docstring"="_LV_(Tick Count (ms),[],[0])"}}, {"module"="pyVI.functions.lvTimeFunctions", "short name"="lvTiming", "docstrings"={"type"="class", "name"="wait", "docstring"="_LV_(Wait (ms),[0],[0])"}}, {"module"="pyVI.functions.lvTimeFunctions", "short name"="lvTiming", "docstrings"={"type"="class", "name"="waitUntilNextMsMultiple", "docstring"="_LV_(Wait Until Next ms Multiple,[0],[0])"}}, {"module"="pyVI.functions.lvTimeFunctions", "short name"="lvTiming", "docstrings"={"type"="class", "name"="getDateTimeString", "docstring"="_LV_(Get Date/Time String,[1,2,0],[1,0])"}}, {"module"="pyVI.functions.lvTimeFunctions", "short name"="lvTiming", "docstrings"={"type"="class", "name"="formatDateTimeString", "docstring"="_LV_(Format Date/Time String,[1,2,0],[0])"}}, {"module"="pyVI.functions.lvTimeFunctions", "short name"="lvTiming", "docstrings"={"type"="class", "name"="secondsToDateTime", "docstring"="_LV_(Seconds To Date/Time,[1,0],[0])"}}, {"module"="pyVI.functions.lvTimeFunctions", "short name"="lvTiming", "docstrings"={"type"="class", "name"="dateTimeToSeconds", "docstring"="_LV_(Date/Time To Seconds,[1,0],[0])"}}, {"module"="pyVI.functions.lvTimeFunctions", "short name"="lvTiming", "docstrings"={"type"="class", "name"="GetDateTimeInSeconds", "docstring"="_LV_(Get Date/Time In Seconds,[],[0])"}}, {"module"="pyVI.functions.lvTrigFunctions", "short name"="lvTrig", "docstrings"={"type"="class", "name"="Sine", "docstring"="_LV_(Sine,[0],[0])"}}, {"module"="pyVI.functions.lvTrigFunctions", "short name"="lvTrig", "docstrings"={"type"="class", "name"="Cosine", "docstring"="_LV_(Cosine,[0],[0])"}}, {"module"="pyVI.functions.lvTrigFunctions", "short name"="lvTrig", "docstrings"={"type"="class", "name"="Tangent", "docstring"="_LV_(Tangent,[0],[0])"}}, {"module"="pyVI.functions.lvTrigFunctions", "short name"="lvTrig", "docstrings"={"type"="class", "name"="Arcsine", "docstring"="_LV_(Inverse Sine,[0],[0])"}}, {"module"="pyVI.functions.lvTrigFunctions", "short name"="lvTrig", "docstrings"={"type"="class", "name"="Arccosine", "docstring"="_LV_(Inverse Cosine,[0],[0])"}}, {"module"="pyVI.functions.lvTrigFunctions", "short name"="lvTrig", "docstrings"={"type"="class", "name"="Arctangent", "docstring"="_LV_(Inverse Tangent,[0],[0])"}}, {"module"="pyVI.functions.lvTrigFunctions", "short name"="lvTrig", "docstrings"={"type"="class", "name"="Arctangent2", "docstring"="_LV_(Inverse Tangent (2 Input),[0,1],[0])"}}, {"module"="pyVI.functions.lvTrigFunctions", "short name"="lvTrig", "docstrings"={"type"="class", "name"="Secant", "docstring"="_LV_(Secant,[0],[0])"}}, {"module"="pyVI.functions.lvTrigFunctions", "short name"="lvTrig", "docstrings"={"type"="class", "name"="Arcsecant", "docstring"="_LV_(Inverse Secant,[0],[0])"}}, {"module"="pyVI.functions.lvTrigFunctions", "short name"="lvTrig", "docstrings"={"type"="class", "name"="Cosecant", "docstring"="_LV_(Cosecant,[0],[0])"}}, {"module"="pyVI.functions.lvTrigFunctions", "short name"="lvTrig", "docstrings"={"type"="class", "name"="Arccosecant", "docstring"="_LV_(Inverse Cosecant,[0],[0])"}}, {"module"="pyVI.functions.lvTrigFunctions", "short name"="lvTrig", "docstrings"={"type"="class", "name"="Cotangent", "docstring"="_LV_(Cotangent,[0],[0])"}}, {"module"="pyVI.functions.lvTrigFunctions", "short name"="lvTrig", "docstrings"={"type"="class", "name"="Arccotangent", "docstring"="_LV_(Inverse Cotangent,[0],[0])"}}, {"module"="pyVI.functions.lvTrigFunctions", "short name"="lvTrig", "docstrings"={"type"="class", "name"="Sinc", "docstring"="_LV_(Sinc,[0],[0])"}}, {"module"="pyVI.functions.lvTrigFunctions", "short name"="lvTrig", "docstrings"={"type"="class", "name"="Sine_and_cosine", "docstring"="_LV_(Sine & Cosine,[0],[0,1])"}}, {"module"="pyVI.functions.lvVisa", "short name"="lvVisa", "docstrings"={"type"="class", "name"="ConfigureSerialPort", "docstring"="_LV_(VISA Configure Serial Port (Instr).vi,[0,4,5,8,6,1,3,2,9,7],[0,1])"}}, {"module"="pyVI.functions.lvVisa", "short name"="lvVisa", "docstrings"={"type"="class", "name"="ConfigureSerialPort2", "docstring"="_LV_(VISA Configure Serial Port (Serial Instr).vi,[0,4,5,8,6,1,3,2,9,7],[0,1])"}}, {"module"="pyVI.functions.lvVisa", "short name"="lvVisa", "docstrings"={"type"="class", "name"="VisaRead", "docstring"="_LV_(VISA Read,[2,1,0],[3,2,1,0])"}}, {"module"="pyVI.functions.lvVisa", "short name"="lvVisa", "docstrings"={"type"="class", "name"="VisaWrite", "docstring"="_LV_(VISA Write,[2,1,0],[2,1,0])"}}, {"module"="pyVI.functions.lvVisa", "short name"="lvVisa", "docstrings"={"type"="class", "name"="VisaClose", "docstring"="_LV_(VISA Close,[1,0],[0])"}}, {"module"="pyVI.functions.lvVisa", "short name"="lvVisa", "docstrings"={"type"="class", "name"="VisaSerialBreak", "docstring"="_LV_(VISA Serial Break (Serial Instr).vi,[2,1,0],[1,0])"}}, {"module"="pyVI.RasPi.lvConsole", "short name"="lvConsole", "docstrings"={"type"="class", "name"="ConsolePrint", "docstring"="_LV_(Console.lvlib:Print.vi,[0],[])"}}, {"module"="pyVI.RasPi.lvConsole", "short name"="lvConsole", "docstrings"={"type"="class", "name"="ConsoleInput", "docstring"="_LV_(Console.lvlib:UserInput.vi,[0],[0])"}}, {"module"="pyVI.RasPi.lvGPIO", "short name"="lvGPIO", "docstrings"={"type"="class", "name"="AddEventDetect", "docstring"="_LV_(GPIO.lvlib:AddEventDetect.vi,[2,0,1,3],[1,0])"}}, {"module"="pyVI.RasPi.lvGPIO", "short name"="lvGPIO", "docstrings"={"type"="class", "name"="ConfigureChannel", "docstring"="_LV_(GPIO.lvlib:ConfigureChannel.vi,[3,1,2,0,4],[0])"}}, {"module"="pyVI.RasPi.lvGPIO", "short name"="lvGPIO", "docstrings"={"type"="class", "name"="ConfigureChannels", "docstring"="_LV_(GPIO.lvlib:ConfigureChannels.vi,[3,1,2,0,4],[0])"}}, {"module"="pyVI.RasPi.lvGPIO", "short name"="lvGPIO", "docstrings"={"type"="class", "name"="EventDetected", "docstring"="_LV_(GPIO.lvlib:EventDetected.vi,[0,1],[1,0])"}}, {"module"="pyVI.RasPi.lvGPIO", "short name"="lvGPIO", "docstrings"={"type"="class", "name"="GetPinNumbering", "docstring"="_LV_(GPIO.lvlib:GetPinNumbering.vi,[0],[1,0])"}}, {"module"="pyVI.RasPi.lvGPIO", "short name"="lvGPIO", "docstrings"={"type"="class", "name"="ReadChannel", "docstring"="_LV_(GPIO.lvlib:ReadChannel.vi,[0,1],[1,0])"}}, {"module"="pyVI.RasPi.lvGPIO", "short name"="lvGPIO", "docstrings"={"type"="class", "name"="RemoveEventDetect", "docstring"="_LV_(GPIO.lvlib:RemoveEventDetect.vi,[0,1],[0])"}}, {"module"="pyVI.RasPi.lvGPIO", "short name"="lvGPIO", "docstrings"={"type"="class", "name"="SetPinNumbering", "docstring"="_LV_(GPIO.lvlib:SetPinNumbering.vi,[0,1],[0])"}}, {"module"="pyVI.RasPi.lvGPIO", "short name"="lvGPIO", "docstrings"={"type"="class", "name"="WaitForEdge_SingleChannel", "docstring"="_LV_(GPIO.lvlib:WaitForEdge_SingleChannel.vi,[3,1,0,2,4],[1,0])"}}, {"module"="pyVI.RasPi.lvGPIO", "short name"="lvGPIO", "docstrings"={"type"="class", "name"="WaitForEdge_MultipleChannels", "docstring"="_LV_(GPIO.lvlib:WaitForEdge_MultipleChannels.vi,[3,1,0,2,4],[1,0])"}}, {"module"="pyVI.RasPi.lvGPIO", "short name"="lvGPIO", "docstrings"={"type"="class", "name"="WriteChannel", "docstring"="_LV_(GPIO.lvlib:WriteChannel.vi,[1,0,2],[0])"}}, {"module"="pyVI.RasPi.lvGPIO", "short name"="lvGPIO", "docstrings"={"type"="class", "name"="WriteChannels_MultipleValues", "docstring"="_LV_(GPIO.lvlib:WriteChannels_MultipleValues.vi,[1,0,2],[0])"}}, {"module"="pyVI.RasPi.lvGPIO", "short name"="lvGPIO", "docstrings"={"type"="class", "name"="WriteChannels_SingleValue", "docstring"="_LV_(GPIO.lvlib:WriteChannels_SingleValue.vi,[1,0,2],[0])"}}, {"module"="pyVI.RasPi.lvGPIO", "short name"="lvGPIO", "docstrings"={"type"="class", "name"="ConfigurePWM", "docstring"="_LV_(GPIO.lvlib:ConfigurePWM.vi,[4,3,5],[0])"}}, {"module"="pyVI.RasPi.lvGPIO", "short name"="lvGPIO", "docstrings"={"type"="class", "name"="StartPWM", "docstring"="_LV_(GPIO.lvlib:StartPWM.vi,[4,3,5],[0])"}}, {"module"="pyVI.RasPi.lvGPIO", "short name"="lvGPIO", "docstrings"={"type"="class", "name"="StopPWM", "docstring"="_LV_(GPIO.lvlib:StopPWM.vi,[4,5],[0])"}}, {"module"="pyVI.RasPi.lvGPIO", "short name"="lvGPIO", "docstrings"={"type"="class", "name"="ChangeFrequency", "docstring"="_LV_(GPIO.lvlib:ChangePWMFrequency.vi,[4,3,5],[0])"}}, {"module"="pyVI.RasPi.lvGPIO", "short name"="lvGPIO", "docstrings"={"type"="class", "name"="ChangeDutyCycle", "docstring"="_LV_(GPIO.lvlib:ChangePWMDutyCycle.vi,[4,3,5],[0])"}}, {"module"="pyVI.RasPi.lvI2C", "short name"="lvI2C", "docstrings"={"type"="class", "name"="I2C_Open", "docstring"="_LV_(GPIO.lvlib:I2C_Open.vi,[0,1],[0])"}}, {"module"="pyVI.RasPi.lvI2C", "short name"="lvI2C", "docstrings"={"type"="class", "name"="I2C_Close", "docstring"="_LV_(GPIO.lvlib:I2C_Close.vi,[0,1],[0])"}}, {"module"="pyVI.RasPi.lvI2C", "short name"="lvI2C", "docstrings"={"type"="class", "name"="I2C_Busses", "docstring"="_LV_(GPIO.lvlib:I2C_Busses.vi,[0],[1,0])"}}, {"module"="pyVI.RasPi.lvI2C", "short name"="lvI2C", "docstrings"={"type"="class", "name"="I2C_Detect", "docstring"="_LV_(GPIO.lvlib:I2C_Detect.vi,[0,1],[1,0])"}}, {"module"="pyVI.RasPi.lvI2C", "short name"="lvI2C", "docstrings"={"type"="class", "name"="I2C_ReadBlockData", "docstring"="_LV_(GPIO.lvlib:I2C_ReadBlockData.vi,[0,2,1,4,3],[1,0])"}}, {"module"="pyVI.RasPi.lvI2C", "short name"="lvI2C", "docstrings"={"type"="class", "name"="I2C_ReadByte", "docstring"="_LV_(GPIO.lvlib:I2C_ReadByte.vi,[0,1,2],[1,0])"}}, {"module"="pyVI.RasPi.lvI2C", "short name"="lvI2C", "docstrings"={"type"="class", "name"="I2C_ReadByteData", "docstring"="_LV_(GPIO.lvlib:I2C_ReadByteData.vi,[0,2,1,3],[1,0])"}}, {"module"="pyVI.RasPi.lvI2C", "short name"="lvI2C", "docstrings"={"type"="class", "name"="I2C_ReadWordData", "docstring"="_LV_(GPIO.lvlib:I2C_ReadWordData.vi,[0,2,1,3],[1,0])"}}, {"module"="pyVI.RasPi.lvI2C", "short name"="lvI2C", "docstrings"={"type"="class", "name"="I2C_WriteByte", "docstring"="_LV_(GPIO.lvlib:I2C_WriteByte.vi,[1,2,0,3],[0])"}}, {"module"="pyVI.RasPi.lvI2C", "short name"="lvI2C", "docstrings"={"type"="class", "name"="I2C_WriteBlockData", "docstring"="_LV_(GPIO.lvlib:I2C_WriteBlockData.vi,[1,3,2,0,4],[0])"}}, {"module"="pyVI.RasPi.lvI2C", "short name"="lvI2C", "docstrings"={"type"="class", "name"="I2C_WriteByteData", "docstring"="_LV_(GPIO.lvlib:I2C_WriteByteData.vi,[1,3,2,0,4],[0])"}}, {"module"="pyVI.RasPi.lvI2C", "short name"="lvI2C", "docstrings"={"type"="class", "name"="I2C_WriteWordData", "docstring"="_LV_(GPIO.lvlib:I2C_WriteWordData.vi,[1,3,2,0,4],[0])"}}, {"module"="pyVI.RasPi.lvI2C", "short name"="lvI2C", "docstrings"={"type"="class", "name"="I2C_WriteQuick", "docstring"="_LV_(GPIO.lvlib:I2C_WriteQuick.vi,[0,1,2],[0])"}}, {"module"="pyVI.RasPi.lvSPI", "short name"="lvSPI", "docstrings"={"type"="class", "name"="SPI_Open", "docstring"="_LV_(GPIO.lvlib:SPI_Open.vi,[1,0,2],[0])"}}, {"module"="pyVI.RasPi.lvSPI", "short name"="lvSPI", "docstrings"={"type"="class", "name"="SPI_Close", "docstring"="_LV_(GPIO.lvlib:SPI_Close.vi,[1,0,2],[0])"}}, {"module"="pyVI.RasPi.lvSPI", "short name"="lvSPI", "docstrings"={"type"="class", "name"="SPI_GetChipSelectActiveState", "docstring"="_LV_(GPIO.lvlib:SPI_GetChipSelectActiveState.vi,[1,0,2],[1,0])"}}, {"module"="pyVI.RasPi.lvSPI", "short name"="lvSPI", "docstrings"={"type"="class", "name"="SPI_GetMaxSpeed", "docstring"="_LV_(GPIO.lvlib:SPI_GetMaxSpeed.vi,[1,0,2],[1,0])"}}, {"module"="pyVI.RasPi.lvSPI", "short name"="lvSPI", "docstrings"={"type"="class", "name"="SPI_GetMode", "docstring"="_LV_(GPIO.lvlib:SPI_GetMode.vi,[1,0,2],[1,0])"}}, {"module"="pyVI.RasPi.lvSPI", "short name"="lvSPI", "docstrings"={"type"="class", "name"="SPI_GetThreeWire", "docstring"="_LV_(GPIO.lvlib:SPI_GetThreeWire.vi,[1,0,2],[1,0])"}}, {"module"="pyVI.RasPi.lvSPI", "short name"="lvSPI", "docstrings"={"type"="class", "name"="SPI_ReadBytes", "docstring"="_LV_(GPIO.lvlib:SPI_ReadBytes.vi,[2,0,1,3],[1,0])"}}, {"module"="pyVI.RasPi.lvSPI", "short name"="lvSPI", "docstrings"={"type"="class", "name"="SPI_SetChipSelectActiveState", "docstring"="_LV_(GPIO.lvlib:SPI_SetChipSelectActiveState.vi,[2,0,1,3],[0])"}}, {"module"="pyVI.RasPi.lvSPI", "short name"="lvSPI", "docstrings"={"type"="class", "name"="SPI_SetMaxSpeed", "docstring"="_LV_(GPIO.lvlib:SPI_SetMaxSpeed.vi,[2,0,1,3],[0])"}}, {"module"="pyVI.RasPi.lvSPI", "short name"="lvSPI", "docstrings"={"type"="class", "name"="SPI_SetMode", "docstring"="_LV_(GPIO.lvlib:SPI_SetMode.vi,[2,0,1,3],[0])"}}, {"module"="pyVI.RasPi.lvSPI", "short name"="lvSPI", "docstrings"={"type"="class", "name"="SPI_SetThreeWire", "docstring"="_LV_(GPIO.lvlib:SPI_SetThreeWire.vi,[2,0,1,3],[0])"}}, {"module"="pyVI.RasPi.lvSPI", "short name"="lvSPI", "docstrings"={"type"="class", "name"="SPI_Transaction", "docstring"="_LV_(GPIO.lvlib:SPI_Transaction.vi,[2,0,1,5,4,3],[1,0])"}}, {"module"="pyVI.RasPi.lvSPI", "short name"="lvSPI", "docstrings"={"type"="class", "name"="SPI_Transaction2", "docstring"="_LV_(GPIO.lvlib:SPI_Transaction2.vi,[2,0,1,5,4,3],[1,0])"}}, {"module"="pyVI.RasPi.lvSPI", "short name"="lvSPI", "docstrings"={"type"="class", "name"="SPI_WriteBytes", "docstring"="_LV_(GPIO.lvlib:SPI_WriteBytes.vi,[2,0,1,3],[0])"}}, {"module"="pyVI.RasPi.REC4", "short name"="REC4", "docstrings"={"type"="class", "name"="REC4_Open", "docstring"="_LV_(REC4.lvlib:REC4_Open.vi,[1,0],[1,0])"}}, {"module"="pyVI.RasPi.REC4", "short name"="REC4", "docstrings"={"type"="class", "name"="REC4_ConfigureIO", "docstring"="_LV_(REC4.lvlib:REC4_ConfigureIO.vi,[2,0,1],[1,0])"}}, {"module"="pyVI.RasPi.REC4", "short name"="REC4", "docstrings"={"type"="class", "name"="REC4_Close", "docstring"="_LV_(REC4.lvlib:REC4_Close.vi,[1,0],[0])"}}]) -> (3 "supported functions":variant)   [LabVIEW 2014, in "Python Functions.lvlib"]
uses:
  Python Functions.lvlib
  FunctionsTD.ctl
  DocstringTD.ctl
  Classes/PythonFunction/PythonFunction.lvclass/PythonFunction.ctl
  Classes/PythonFunction/PythonFunction.lvclass
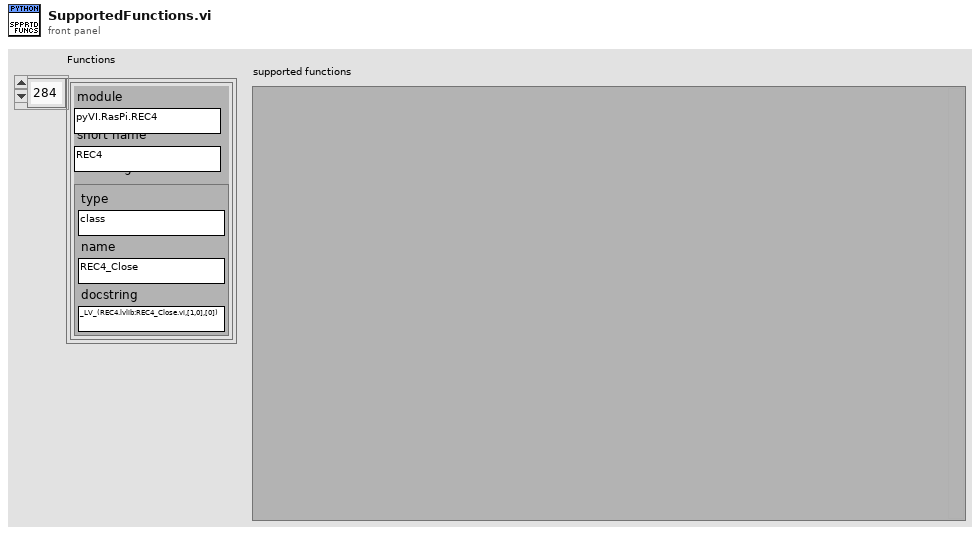
[diagram p1: front panel]
types:
  T1 = typedef "Python Functions.lvlib/FunctionsTD.ctl" = cluster{"module":string, "short name":string, "docstrings":T2}[]
  T2 = typedef "Python Functions.lvlib/DocstringTD.ctl" = cluster{"type":string, "name":string, "docstring":string}
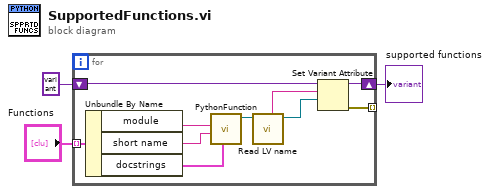
[diagram p0: block diagram]
diagram:
  n1 = for {
    shift-right: [w12] -> w1
    shift-left: variant -> [w11]
    tunnel: [w8] -> _ mode=indexing
    tunnel: "Functions" -> [w7] mode=indexing
    n2 = Unbundle By Name(w7) -> ("module"=w4:string, "short name"=w5:string, "docstrings"=w6:T2)
    n3 = call "PythonFunction.vi"("info"=w6, "Python module  name"=w5, "Python module"=w4) -> ("PythonFunction out"=w13:refnum<class "PythonFunction.lvclass">)  [unwired: 8 in]
    n4 = call "Read LV name.vi"("PythonFunction in"=w13) -> ("PythonFunction out"=w9:refnum<class "PythonFunction.lvclass">, "LV name"=w10:string)  [unwired: 7 in]
    n5 = Set Variant Attribute(Variant=w11, name=w10, value=w9) -> (Variant out=w12:variant, error out=w8:errorcluster)  [unwired: 1 in, 1 out]
  }
  "supported functions" <- w1
